vi "Lookup Query Parameter.vi"(8 "error in (no error)":errorcluster, 10 "Name":string, 11 "URI in":refnum<class "URI.lvclass">) -> (0 "error out":errorcluster, 1 "Found":bool, 2 "Value":string, 3 "URI out":refnum<class "URI.lvclass">)   [LabVIEW 2020, in "URI.lvclass"]
uses:
  URI.lvclass
  URI.lvclass/URI.ctl
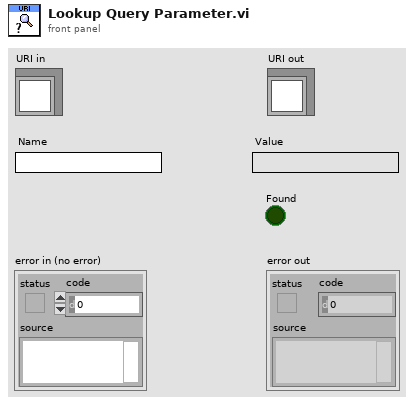
[diagram p1: front panel]
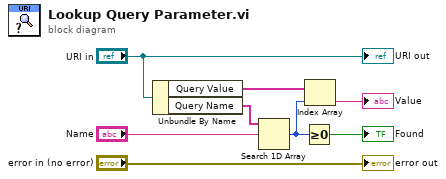
[diagram p0: block diagram]
diagram:
  n1 = Unbundle By Name("URI in") -> ("Query Value"=w4:string[], "Query Name"=w6:string[])
  n2 = Search 1D Array(1D array=w6, element="Name") -> (index of element=w2:i32)  [unwired: 1 in]
  n3 = Greater Or Equal To 0?(x=w2) -> (x >= 0?=→"Found":bool)
  n4 = Index Array(array=w4, index=w2) -> (element=→"Value":string)
  "error out" <- "error in (no error)"
  "URI out" <- "URI in"
